vi "Set 2D Next Vector_IS.vi"(0 "Coordinate System":u16(ring) items=["Cartesian", "Polar"], 1 "Magnetic Field Units":u16(ring) items=["kG", "Tesla"], 3 "Input Vector":string[](array[string]), 4 "User defined Ramp Rate (T/min)":dbl format="%.3f", 5 "Magnitude Limit (kG)":dbl format="%.3f", 7 "Y-Axis Communications Config":T4={"GPIB address"=22, "GPIB bus"=0, "connection ID"=refnum, "IP"="192.168.2.200", "Active Comm Interface"=0, "Serial Port"="", "Programmer Type"=0} {"Programmer Type" items=["Model 430", "Model 420"]; "Active Comm Interface" items=["TCP/IP (Model 430 Only)", "RS232", "IEEE488"]}, 8 "sweep parameter":T1=enum."magnetic field", 9 "Z-Axis Communications Config":T4={"GPIB address"=22, "GPIB bus"=0, "connection ID"=refnum, "IP"="192.168.2.200", "Active Comm Interface"=0, "Serial Port"="", "Programmer Type"=0} {"Programmer Type" items=["Model 430", "Model 420"]; "Active Comm Interface" items=["TCP/IP (Model 430 Only)", "RS232", "IEEE488"]}, 12 "Delta phi (deg)":dbl=0.5 format="%.3f", 13 "Delta H (mT)":dbl=0.5 format="%.3f", 14 "User defined Ramp Rate?":bool, 17 "Max Ramp Rate - Y Axis (A/s)":dbl format="%.3f", 18 "const phi?":bool, 20 "error in":T3, 21 "Max Ramp Rate - Z Axis (A/s)":dbl format="%.3f") -> (15 "Y-Axis Ramp Rate (T/min)":dbl format="%.3f", 16 "Within Limits?":bool, 23 "Ramp Rate along Vector (T/min)":dbl, 24 "Z-Axis Ramp Rate (T/min)":dbl format="%.3f", 25 "All Instruments Responded?":bool, 27 "error out":T3)   [LabVIEW 2013]
uses:
  AMI reading polar field.ctl
  measurement/measurement sweep parameter.ctl
  app/app global state actions.ctl
panel:
  out "Current Magnetic\nField\n(430 TCP reading)":T2 {"phi (deg)" format="%#_3g"}
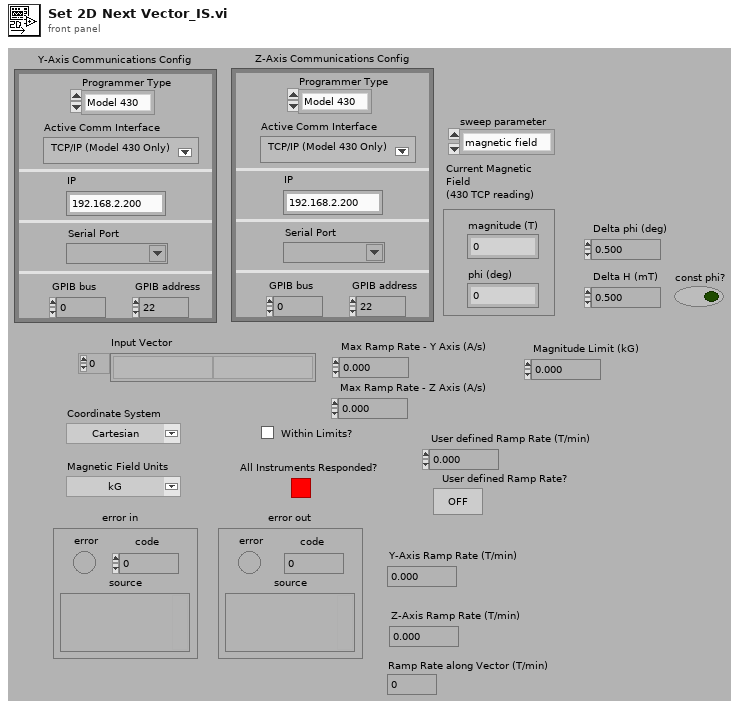
[diagram p1: front panel]
types:
  T1 = typedef "measurement sweep parameter.ctl" = enum16{"angle", "magnetic field"}
  T2 = typedef "AMI reading polar field.ctl" = cluster{"magnitude (T)":dbl, "phi (deg)":dbl}
  T3 = cluster{"error":bool, "code":i32, "source":string}
  T4 = cluster{"GPIB address":i16, "GPIB bus":i16, "connection ID":refnum<k5>, "IP":string, "Active Comm Interface":u16, "Serial Port":refnum<visa-resource-name>, "Programmer Type":u16}
  T5 = typedef "app global state actions.ctl" = enum16{"set field reached", "get cluster", "set cluster", "set current sweep", "set field value", "set 430 TCP reading", "set ramping", "set sweeping", "append log", "clear log", "set finished"}
  T6 = typedef "app global state control.ctl" = cluster{"current field value":T7, "field ramping":bool, "vna sweeping":bool, "Log Messages":string, "current sweep":T8, "measurement finished":bool, "Current Magnetic Field\n(430 TCP reading)":cluster{"magnitude (T)":dbl, "phi (deg)":dbl}, "field was reached":bool}
  T7 = typedef "magnet polar field.ctl" = cluster{"magnitude":dbl, "phi":dbl, "theta":dbl}
  T8 = typedef "measconfig cluster.ctl" = cluster{"sweep parameter":T1, "sweep start":dbl, "sweep stop":dbl, "sweep increment":dbl, "temperature":dbl, "path":path, "magnet initial":T7, "magnet reference":T7, "const phi?":bool, "delta phi (deg)":dbl, "delta H (mT)":dbl}
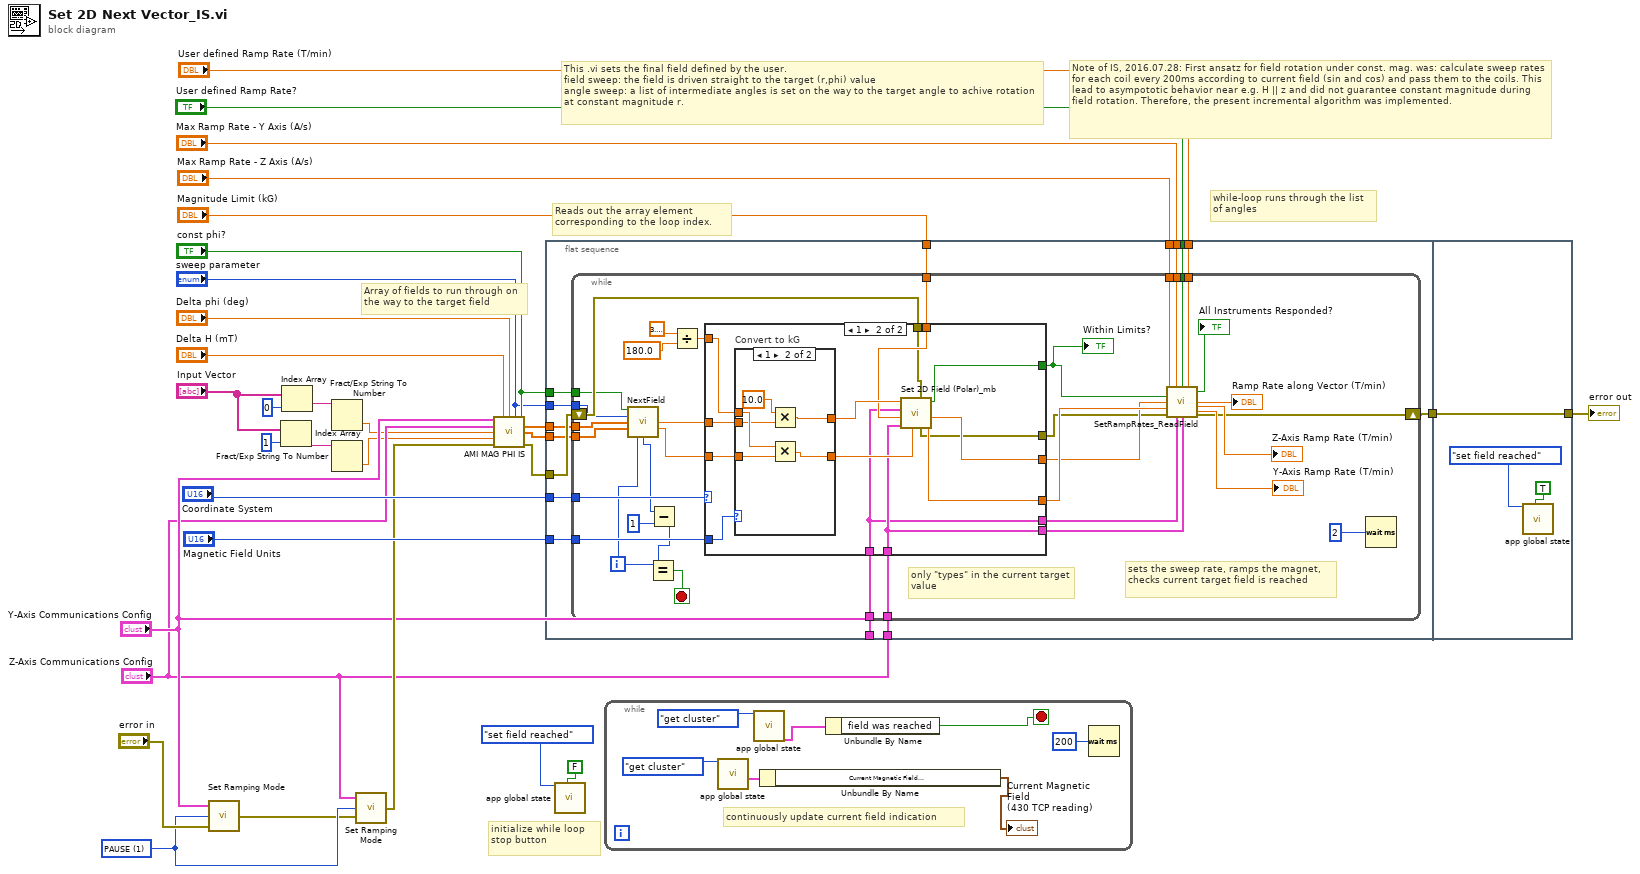
[diagram p0: block diagram]
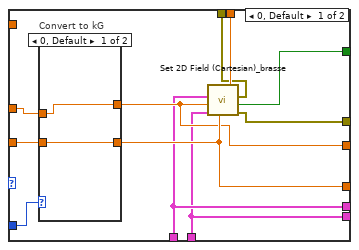
[diagram p2: hidden frame]
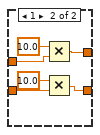
[diagram p3: hidden frame]
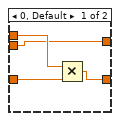
[diagram p4: hidden frame]
diagram:
  w24 = u16 1 items=["RAMP", "PAUSE", "MANUAL UP", "MANUAL DOWN", "ZERO"] ("Ramping Mode")
  # "Reads out the array element corresponding to the loop index."
  # "Note of IS, 2016.07.28: First ansatz for field rotation under const. mag. was: calculate sweep rates for each coil every 200ms according to current field (sin and cos) and pass them to the coils. This lead to asympototic behavior near e.g. H || z and did not guarantee constant magnitude during field rotation. Therefore, the present incremental algorithm was implemented."
  # "while-loop runs through the list\nof angles"
  # "Array of fields to run through on the way to the target field"
  # "initialize while loop\nstop button"
  # "This .vi sets the final field defined by the user.\nfield sweep: the field is driven straight to the target (r,phi) value\nangle sweep: a list of intermediate angles is set on the way to the target angle to achive rotation at constant magnitude r."
  n1 = call <userlib>:"Set Ramping Mode.vi"("error in"="error in", "Ramping Mode"=w24, "Communications Config"="Y-Axis Communications Config") -> ("error out"=w20:T3)
  n2 = Index Array(array="Input Vector", index=1 ("Index")) -> (element=w27:string)
  n3 = Index Array(array="Input Vector", index=0 ("Index")) -> (element=w28:string)
  n4 = Fract/Exp String To Number(string=w28) -> (number=w10:dbl)  [unwired: 3 in, 1 out]
  n5 = Fract/Exp String To Number(string=w27) -> (number=w9:dbl)  [unwired: 3 in, 1 out]
  n6 = call <userlib>:"Set Ramping Mode.vi"("error in"=w20, "Ramping Mode"=w24, "Communications Config"="Z-Axis Communications Config") -> ("error out"=w14:T3)
  n7 = call "AMI MAG PHI IS.vi"("Y-Axis Communications Config"="Y-Axis Communications Config", "delta H (mT)"="Delta H (mT)", "delta phi (deg)"="Delta phi (deg)", "sweep parameter"="sweep parameter", "const phi?"="const phi?", "Z-Axis Communications Config"="Z-Axis Communications Config", "target mag in (T)"=w10, "target phi (deg)"=w9, "error in (no error)"=w14) -> ("target mag out (T)"=w5:dbl[], "phi array (deg)"=w8:dbl[], "error out"=w13:T3)  [unwired: 4 in]
  n8 = flat-sequence {
    tunnel: "Magnetic Field Units" -> [w46]
    tunnel: "Magnitude Limit (kG)" -> [w45]
    tunnel: "Coordinate System" -> [w44]
    tunnel: "User defined Ramp Rate?" -> [w43]
    tunnel: "Max Ramp Rate - Y Axis (A/s)" -> [w42]
    tunnel: "Max Ramp Rate - Z Axis (A/s)" -> [w41]
    tunnel: "User defined Ramp Rate (T/min)" -> [w40]
    tunnel: w8 -> [w35]
    tunnel: w13 -> [w39]
    tunnel: "Y-Axis Communications Config" -> [w38]
    tunnel: "Z-Axis Communications Config" -> [w37]
    tunnel: [w36] -> w15
    tunnel: w5 -> [w34]
    tunnel: "const phi?" -> [w33]
    tunnel: "sweep parameter" -> [w32]
    tunnel: [w128] -> w16
    tunnel: w15 -> [w128]
    frame #0 {
      n9 = while {
        tunnel: w46 -> [w82]
        tunnel: w45 -> [w79]
        tunnel: w44 -> [w78]
        tunnel: w43 -> [w76]
        tunnel: w38 -> [w73]
        tunnel: w37 -> [w72]
        tunnel: w42 -> [w71]
        tunnel: w41 -> [w70]
        tunnel: w40 -> [w65]
        shift-right: [w60] -> w36
        shift-left: w39 -> [w59]
        tunnel: w35 -> [w54]
        tunnel: w34 -> [w55]
        tunnel: w33 -> [w56]
        tunnel: w32 -> [w53]
        i -> [w51]
        stop <- w52 stop-if-true
        # "only \"types\" in the current target value"
        # "sets the sweep rate, ramps the magnet, checks current target field is reached"
        n10 = call "NextField.vi"("const phi?"=w56, "sweep parameter"=w53, "target mag (T)"=w55, "phi array (deg)"=w54, "Loop index"=w51) -> ("Next mag (T)"=w58:dbl, "Next phi (deg)"=w57:dbl, "Loop Count"=w49:i32)  [unwired: 8 in]
        n11 = Subtract(x=w49, y=1) -> (x-y=w48:i32)
        n12 = Equal?(x=w51, y=w48) -> (x = y?=w52:bool)
        n13 = Divide(x=3.141592653589793, y=180.0) -> (x/y=w77:dbl)
        n14 = case shown="1" w78 {
          tunnel: w82 -> [w93 w115]
          tunnel: w57 -> [w92 w114]
          tunnel: w73 -> [w86 w104]
          tunnel: w72 -> [w85 w105]
          tunnel: [w91 w111] -> w69
          tunnel: [w90 w109] -> w75
          tunnel: [w89 w110] -> w74
          tunnel: w77 -> [_ w113]
          tunnel: w79 -> [w88 w107]
          tunnel: [w87 w106] -> w68
          tunnel: [w85 w105] -> w67
          tunnel: [w86 w104] -> w66
          tunnel: w59 -> [w84 w103]
          tunnel: w58 -> [w83 w102]
          frame 0, Default {
            n15 = case "Convert to kG" shown="0, Default" w93 {
              tunnel: w92 -> [w95 w99]
              tunnel: [w94 w98] -> w89
              tunnel: [w95 w97] -> w90
              tunnel: w83 -> [w94 w96]
              frame 0, Default {
              }
              frame 1 {
                n16 = Multiply(x=10.0, y=w96) -> (x*y=w98:dbl)
                n17 = Multiply(x=10.0, y=w99) -> (x*y=w97:dbl)
              }
            }
            n18 = call <userlib>:"Set 2D Field (Cartesian)_brasse.vi"("error in"=w84, "Magnitude Limit (kG)"=w88, "Z-Axis Field (kG)"=w90, "Z-Axis Communications Config"=w85, "Y-Axis Field (kG)"=w89, "Y-Axis Communications Config"=w86) -> ("error out"=w87:T3, "Within Limits?"=w91:bool)  [unwired: 2 in]
          }
          frame 1 {
            n19 = case "Convert to kG" shown="1" w115 {
              tunnel: w114 -> [w118 w125]
              tunnel: [w116 w124] -> w108
              tunnel: [w117 w123] -> w112
              tunnel: w113 -> [w119 w122]
              tunnel: w102 -> [w116 w120]
              frame 0, Default {
                n20 = Multiply(x=w119, y=w118) -> (x*y=w117:dbl)
              }
              frame 1 {
                n21 = Multiply(x=10.0, y=w120) -> (x*y=w124:dbl)
                n22 = Multiply(x=w122, y=w125) -> (x*y=w123:dbl)
              }
            }
            n23 = call <userlib>:"Set 2D Field (Polar)_mb.vi"("error in"=w103, "f (radians)"=w112, "Z-Axis Communications Config"=w105, "Magnitude Limit (kG)"=w107, "Y-Axis Communications Config"=w104, "Field Magnitude r (kG)"=w108) -> ("Z-Axis Field (kG) out"=w109:dbl, "Y-Axis Field (kG)"=w110:dbl, "Within Limits?"=w111:bool, "error out"=w106:T3)  [unwired: 2 in]
          }
        }
        "Within Limits?" <- w69
        n24 = call "SetRampRates_ReadField.vi"("Max Ramp Rate - Z Axis (A/s)"=w70, "Max Ramp Rate - Y Axis (A/s)"=w71, "User defined Ramp Rate (T/min) 2"=w76, "User defined Ramp Rate (T/min)"=w65, "Within Limits?"=w69, "Y-Axis Field (kG)"=w74, "Z-Axis Field (kG) in"=w75, "error in (no error)"=w68, "Y-Axis Communications Config"=w66, "Z-Axis Communications Config"=w67) -> ("All Instruments Responded?"=→"All Instruments Responded?":bool, "Ramp Rate along Vector (T/min)"=→"Ramp Rate along Vector (T/min)":dbl, "Y-Axis Ramp Rate (T/min)"=→"Y-Axis Ramp Rate (T/min)":dbl, "Z-Axis Ramp Rate (T/min)"=→"Z-Axis Ramp Rate (T/min)":dbl, "error out"=w60:T3)  [unwired: 1 out]
        n25 = Wait (ms)(milliseconds to wait=2) -> ()  [unwired: 1 out]
      }
    }
    frame #1 {
      n26 = call "app global state.vi"("action"=app_global_state_actions."set field reached" ("app global state actions"), "field was reached"=TRUE ("measurement finished")) -> ()  [unwired: 17 in, 1 out]
    }
  }
  n27 = call "app global state.vi"("action"=app_global_state_actions."set field reached" ("app global state actions"), "field was reached"=FALSE ("measurement finished")) -> ()  [unwired: 17 in, 1 out]
  n28 = while {
    stop <- w132 stop-if-true
    # "continuously update current field indication"
    n29 = call "app global state.vi"("action"=app_global_state_actions."get cluster" ("app global state actions")) -> ("global state"=w130:T6)  [unwired: 18 in]
    n30 = call "app global state.vi"("action"=app_global_state_actions."get cluster" ("app global state actions")) -> ("global state"=w134:T6)  [unwired: 18 in]
    n31 = Unbundle By Name(w130) -> ("Current Magnetic Field\n(430 TCP reading)"=→"Current Magnetic\nField\n(430 TCP reading)":cluster{"magnitude (T)":dbl, "phi (deg)":dbl})
    n32 = Unbundle By Name(w134) -> ("field was reached"=w132:bool)
    n33 = Wait (ms)(milliseconds to wait=200) -> ()  [unwired: 1 out]
  }
  "error out" <- w16
